vi "IVIS FRET_Sort Image Data.vi"(8 "error in (no error)":errorcluster, 9 "[DA Images]":T1[](array[typedef]), 10 "[AA Images]":T1[](array[typedef]), 11 "[DD Images]":T1[](array[typedef])) -> (0 "error out":errorcluster, 3 "Image Array":T2[](array[typedef]))   [LabVIEW 2021]
uses:
  IVIS FRET_Frame Image Components.ctl
  <vilib>/vision/Image Controls.llb/IMAQ Image.ctl
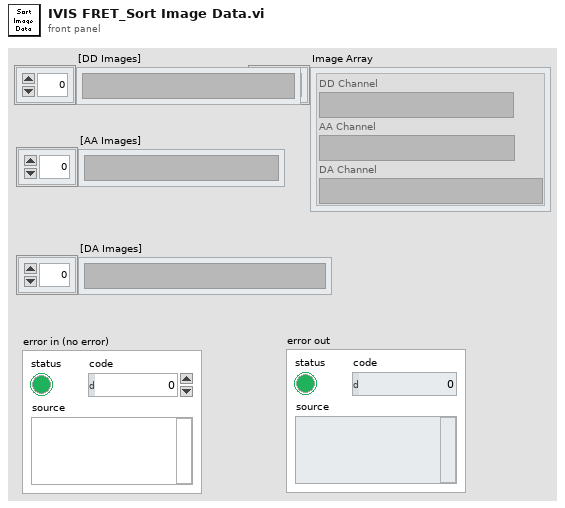
[diagram p1: front panel]
types:
  T1 = typedef "IMAQ Image.ctl" = refnum<image>
  T2 = typedef "IVIS FRET_Frame Image Components.ctl" = cluster{"DD Channel":T1, "AA Channel":T1, "DA Channel":T1}
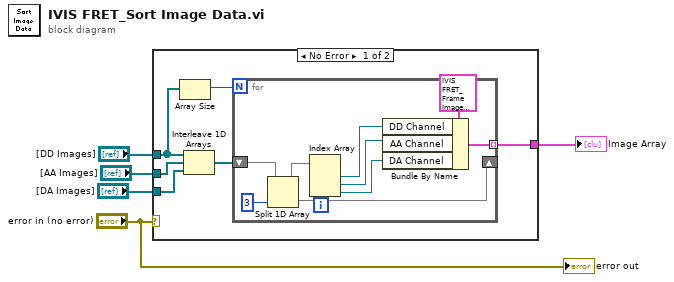
[diagram p0: block diagram]
diagram:
  n1 = case shown="No Error" "error in (no error)" {
    tunnel: [w11 _] -> w5
    tunnel: "[DA Images]" -> [w9 _]
    tunnel: "[AA Images]" -> [w8 _]
    tunnel: "[DD Images]" -> [w7 _]
    frame No Error {
      n2 = Array Size(array=w7) -> (size(s)=w6:i32)
      n3 = Interleave 1D Arrays(w7, w8, w9) -> (w10:T1[])
      n4 = for {
        N: w6 -> [_]
        shift-right: [w18] -> _
        shift-left: w10 -> [w20]
        tunnel: [w12] -> w11 mode=indexing
        n5 = Split 1D Array(array=w20, index=3) -> (first subarray=w16:T1[], second subarray=w18:T1[])
        n6 = Index Array(array=w16) -> (element #1=w15:T1, element #2=w14:T1, element #3=w13:T1)  [unwired: 3 in]
        n7 = Bundle By Name(cluster=T2 {"DD Channel"=refnum, "AA Channel"=refnum, "DA Channel"=refnum}, "DD Channel"=w15, "AA Channel"=w14, "DA Channel"=w13) -> (w12:T2)
      }
    }
    frame Error {
    }
  }
  "Image Array" <- w5
  "error out" <- "error in (no error)"
